vi "Move.vi"(7 "VI":refnum<vi>, 8 "Error":errorcluster, 11 "(FPPos)":refnum<class "Point_FPPos.lvclass">) -> (0 "Error Out":errorcluster, 3 "(FPPos) Out":refnum<class "Point_FPPos.lvclass">, 5 "VI Out":refnum<vi>)   [LabVIEW 2020, in "Point_FPPos.lvclass"]
uses:
  Point_FPPos.lvclass
  Point_FPPos.lvclass/Point_FPPos.ctl
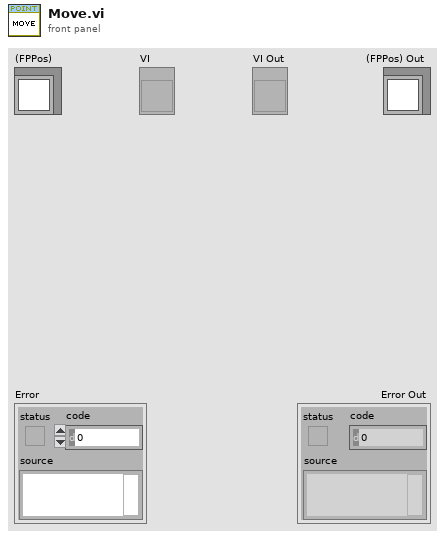
[diagram p1: front panel]
types:
  T1 = typedef "Cluster_Pos_Top Left position.ctl" = cluster{"Left":i16, "Top":i16}
  T2 = typedef "ENUM RB_Pos_Quadrant Position.ctl" = enum32{"LFT-TOP", "MID-TOP", "RGT-TOP", "LFT-CTR", "MID-CTR", "RGT-CTR", "LFT-BOT", "MID-BOT", "RGT-BOT"}
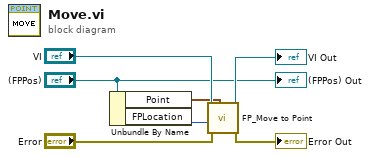
[diagram p0: block diagram]
diagram:
  n1 = Unbundle By Name("(FPPos)") -> ("Point"=w1:T1, "FPLocation"=w2:T2)
  n2 = call "FP_Move to Point.vi"("Target Point"=w1, "Error"="Error", "FP Position"=w2, "VI"="VI") -> ("Error Out"=→"Error Out":errorcluster, "VI Out"=→"VI Out":refnum<vi>)  [unwired: 6 in]
  "(FPPos) Out" <- "(FPPos)"
